vi "Write-Sync-Multiple-TypeResolving-Sensata.vi"() -> ()   [LabVIEW 2020]
doc: "ADS synchronous write example using preconfigured blocks. \n\nThe client writes data synchronously and does wait for the respose from server."
uses:
  <userlib>/Beckhoff-LabVIEW-Interface/_DependsOn/TypeDefs/Low-Levels/Symbol Interface Mode.ctl
  <userlib>/Beckhoff-LabVIEW-Interface/_DependsOn/With TypeResolving/Write Sync Single TypeResolved.vi
panel:
  in  "out_bAsic1CalibrationCompleted_labview":bool=TRUE
  in  "out_bAardvarkBoardError_labview":bool=TRUE
  out "Write Status 3":bool
  out "Has Matched? 3":bool
  out "Write Status 2":bool
  out "Has Matched? 2":bool
  in  "out_strAsic1SerialNo":string="abc1234ser"
  out "Has Matched?":bool
  in  "Symbol file path":path=path "C:/MSDApps/GitHub-Projects/EDP Emotor/Anoop_LabviewTwincatADSTesting/ADS Write Symbols.xml"
  out "Write Status":bool
  # "The example starts with retrieving an\nADS Symbol. The symbol can be selected:\n- Using Symbol file in symbol file path\n- Using Symbol Interface (UI), which is opened automatically if file path is empty.\n\nThe example writes , only once, a string value synchronously to a string variable located in TwinCAT3. Since the  call is synchronous, the example waits for a timeout for an ADS response.\n\nThe example uses TypeResolver to check whether the selected ADS Symbol is of type String or not.\n\nCheck Write status and bHasMached if write has succeeded."
  # "Note: This example is only an illustration of all possible ways how this Product can be used."
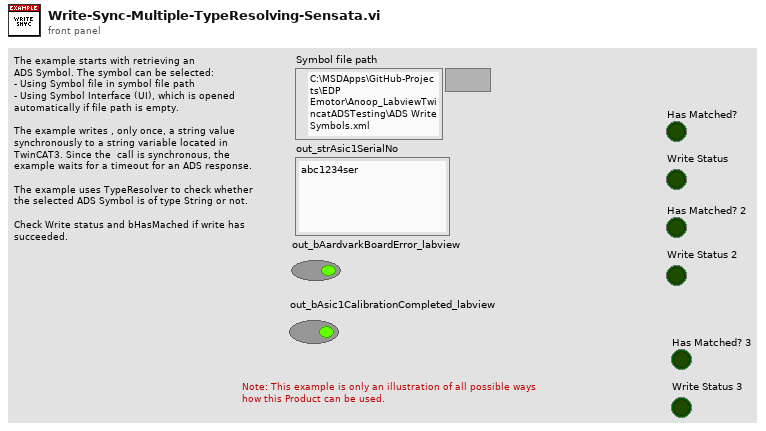
[diagram p1: front panel]
types:
  T1 = cluster{"nVar1":i16, "nVar2":u32, "sVar3":string[]}
  T2 = typedef "Symbol Interface Mode.ctl" = enum16{"Read Only", "Write Only", "Read & Write"}
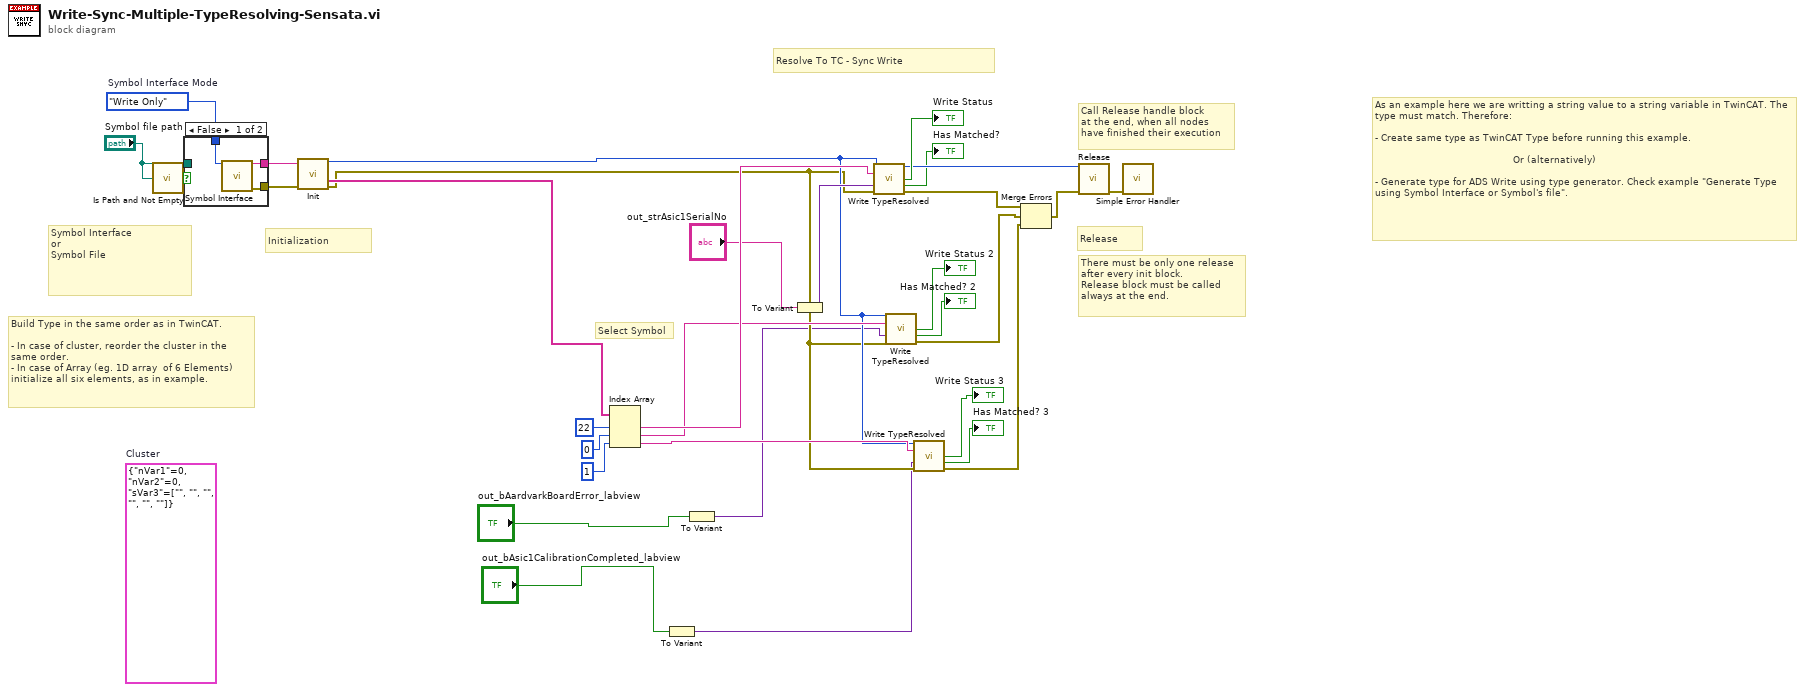
[diagram p0: block diagram]
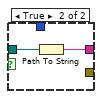
[diagram p2: hidden frame]
diagram:
  (unwired) T1 {"nVar1"=0, "nVar2"=0, "sVar3"=["", "", "", "", "", ""]}  # Cluster
  w20 = Symbol_Interface_Mode."Write Only"  # Symbol Interface Mode
  # "As an example here we are writting a string value to a string variable in TwinCAT. The type must match. Therefore:\n\n- Create same type as TwinCAT Type before running this example. \n                                              \n                                              Or (alternatively)\n\n- Generate type for ADS Write using type generator. Check example \"Generate Type using Symbol Interface or Symbol's file\"."
  # "Build Type in the same order as in TwinCAT.\n\n- In case of cluster, reorder the cluster in the\nsame order.\n- In case of Array (eg. 1D array  of 6 Elements) \ninitialize all six elements, as in example."
  # "Symbol Interface\nor\nSymbol File"
  # "Resolve To TC - Sync Write"
  # "Call Release handle block\nat the end, when all nodes\nhave finished their execution"
  # "There must be only one release\nafter every init block.\nRelease block must be called\nalways at the end."
  # "Select Symbol"
  # "Release"
  # "Initialization"
  n1 = call <vilib>:"Is Path and Not Empty.vi"("path"="Symbol file path") -> ("Is Path and Not Empty?"=w21:bool)  [unwired: 4 in]
  n2 = case shown="False" w21 {
    tunnel: [w35 w37] -> w22
    tunnel: "Symbol file path" -> [_ w36]
    tunnel: [w34 _] -> w23
    tunnel: w20 -> [w33 _]
    frame False {
      n3 = call <userlib>:"Symbol Interface.vi"("Symbol Interface Mode"=w33) -> ("PortInfo"=w35:string, "error out"=w34:errorcluster)  [unwired: 13 in]
    }
    frame True {
      n4 = Path To String(path=w36) -> (string=w37:string)
    }
  }
  n5 = call <userlib>:"Init.vi"("XMLDescription"=w22, "error in (no error)"=w23) -> ("Handle"=w14:u32, "WriteGrpSymbols"=w31:string[], "error out"=w9:errorcluster)  [unwired: 9 in, 2 out]
  n6 = Index Array(array=w31, index #1=22 ("index"), index #2=0 ("index"), index #3=1 ("index")) -> (element #1=w30:string, element #2=w16:string, element #3=w15:string)
  n7 = To Variant(anything="out_bAsic1CalibrationCompleted_labview") -> (Variant=w1:variant)
  n8 = To Variant(anything="out_bAardvarkBoardError_labview") -> (Variant=w2:variant)
  n9 = To Variant(anything="out_strAsic1SerialNo") -> (Variant=w29:variant)
  n10 = call-poly <userlib>:"Write TypeResolved.vi"("Handle"=w14, "SymbolName"=w30, "WData"=w29, "error constant"=w9) -> ("Handle"=w27:u32, "Write Status?"=→"Write Status":bool, "Has Matched?"=→"Has Matched?":bool, "error out"=w8:errorcluster)  [unwired: 8 in]
  n11 = call-poly <userlib>:"Write TypeResolved.vi"("Handle"=w14, "SymbolName"=w16, "WData"=w2, "error constant"=w9) -> ("Write Status?"=→"Write Status 2":bool, "Has Matched?"=→"Has Matched? 2":bool, "error out"=w7:errorcluster)  [unwired: 8 in, 1 out]
  n12 = call-poly <userlib>:"Write TypeResolved.vi"("Handle"=w14, "SymbolName"=w15, "WData"=w1, "error constant"=w9) -> ("Write Status?"=→"Write Status 3":bool, "Has Matched?"=→"Has Matched? 3":bool, "error out"=w6:errorcluster)  [unwired: 8 in, 1 out]
  n13 = Merge Errors(w8, w7, w6) -> (w5:errorcluster)
  n14 = call <userlib>:"Release.vi"("Handle"=w27, "error in (no error)"=w5) -> ("error out"=w19:errorcluster)  [unwired: 13 in]
  n15 = call <vilib>:"Simple Error Handler.vi"("error in (no error)"=w19) -> ()  [unwired: 4 in, 5 out]
